vi "Dipper Fridge Resistance Measurement 1.1.vi"() -> ()   [LabVIEW 2011]
uses:
  <vilib>/express/express arith-compare/Formula/XNode/ExpressFormulaBlockNode.xnode
panel:
  out "Output Power":dbl[unit]
  out "Heater Power (%)":string
  in  "Save":bool
  out "var":i32
  in  "error in (no error) 2":errorcluster
  in  "Output Range":string(combo)
  in  "Heater Power (%)":dbl caption="y"
  out "Heater Type (in Ohm)":string
  out "Heater Current (in %)":string
  out "Heater":bool
  in  "Heater":bool
  out "Boolean":bool
  in  "Power":bool
  in  "Date format (0)":enum16{"short", "long", "abbreviated"}(ring)
  out "Lakeshore":cluster{dbl[], dbl[unit][]}(graph)
  out "Chanel A":cluster{dbl[], dbl[unit][]}(graph)
  out "size (in bytes)":i64
  out "Chanel B":cluster{dbl[], dbl[]}(graph)
  out "Warning":string="Can't be smaller than 1 s"
  in  "File Path":path
  out "current time":timestamp
  out "Number of Data points":i32
  in  "Time delay":u32
  in  "error in (no error)":errorcluster
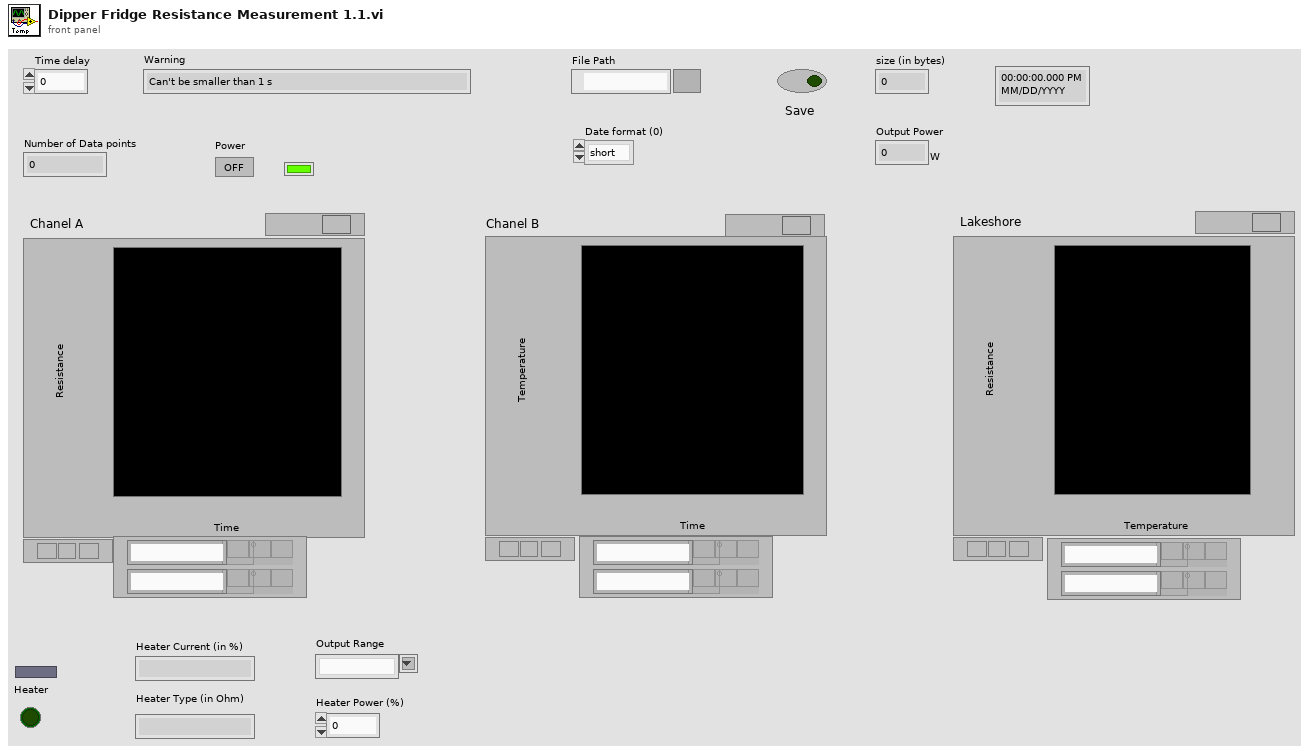
[diagram p1: front panel]
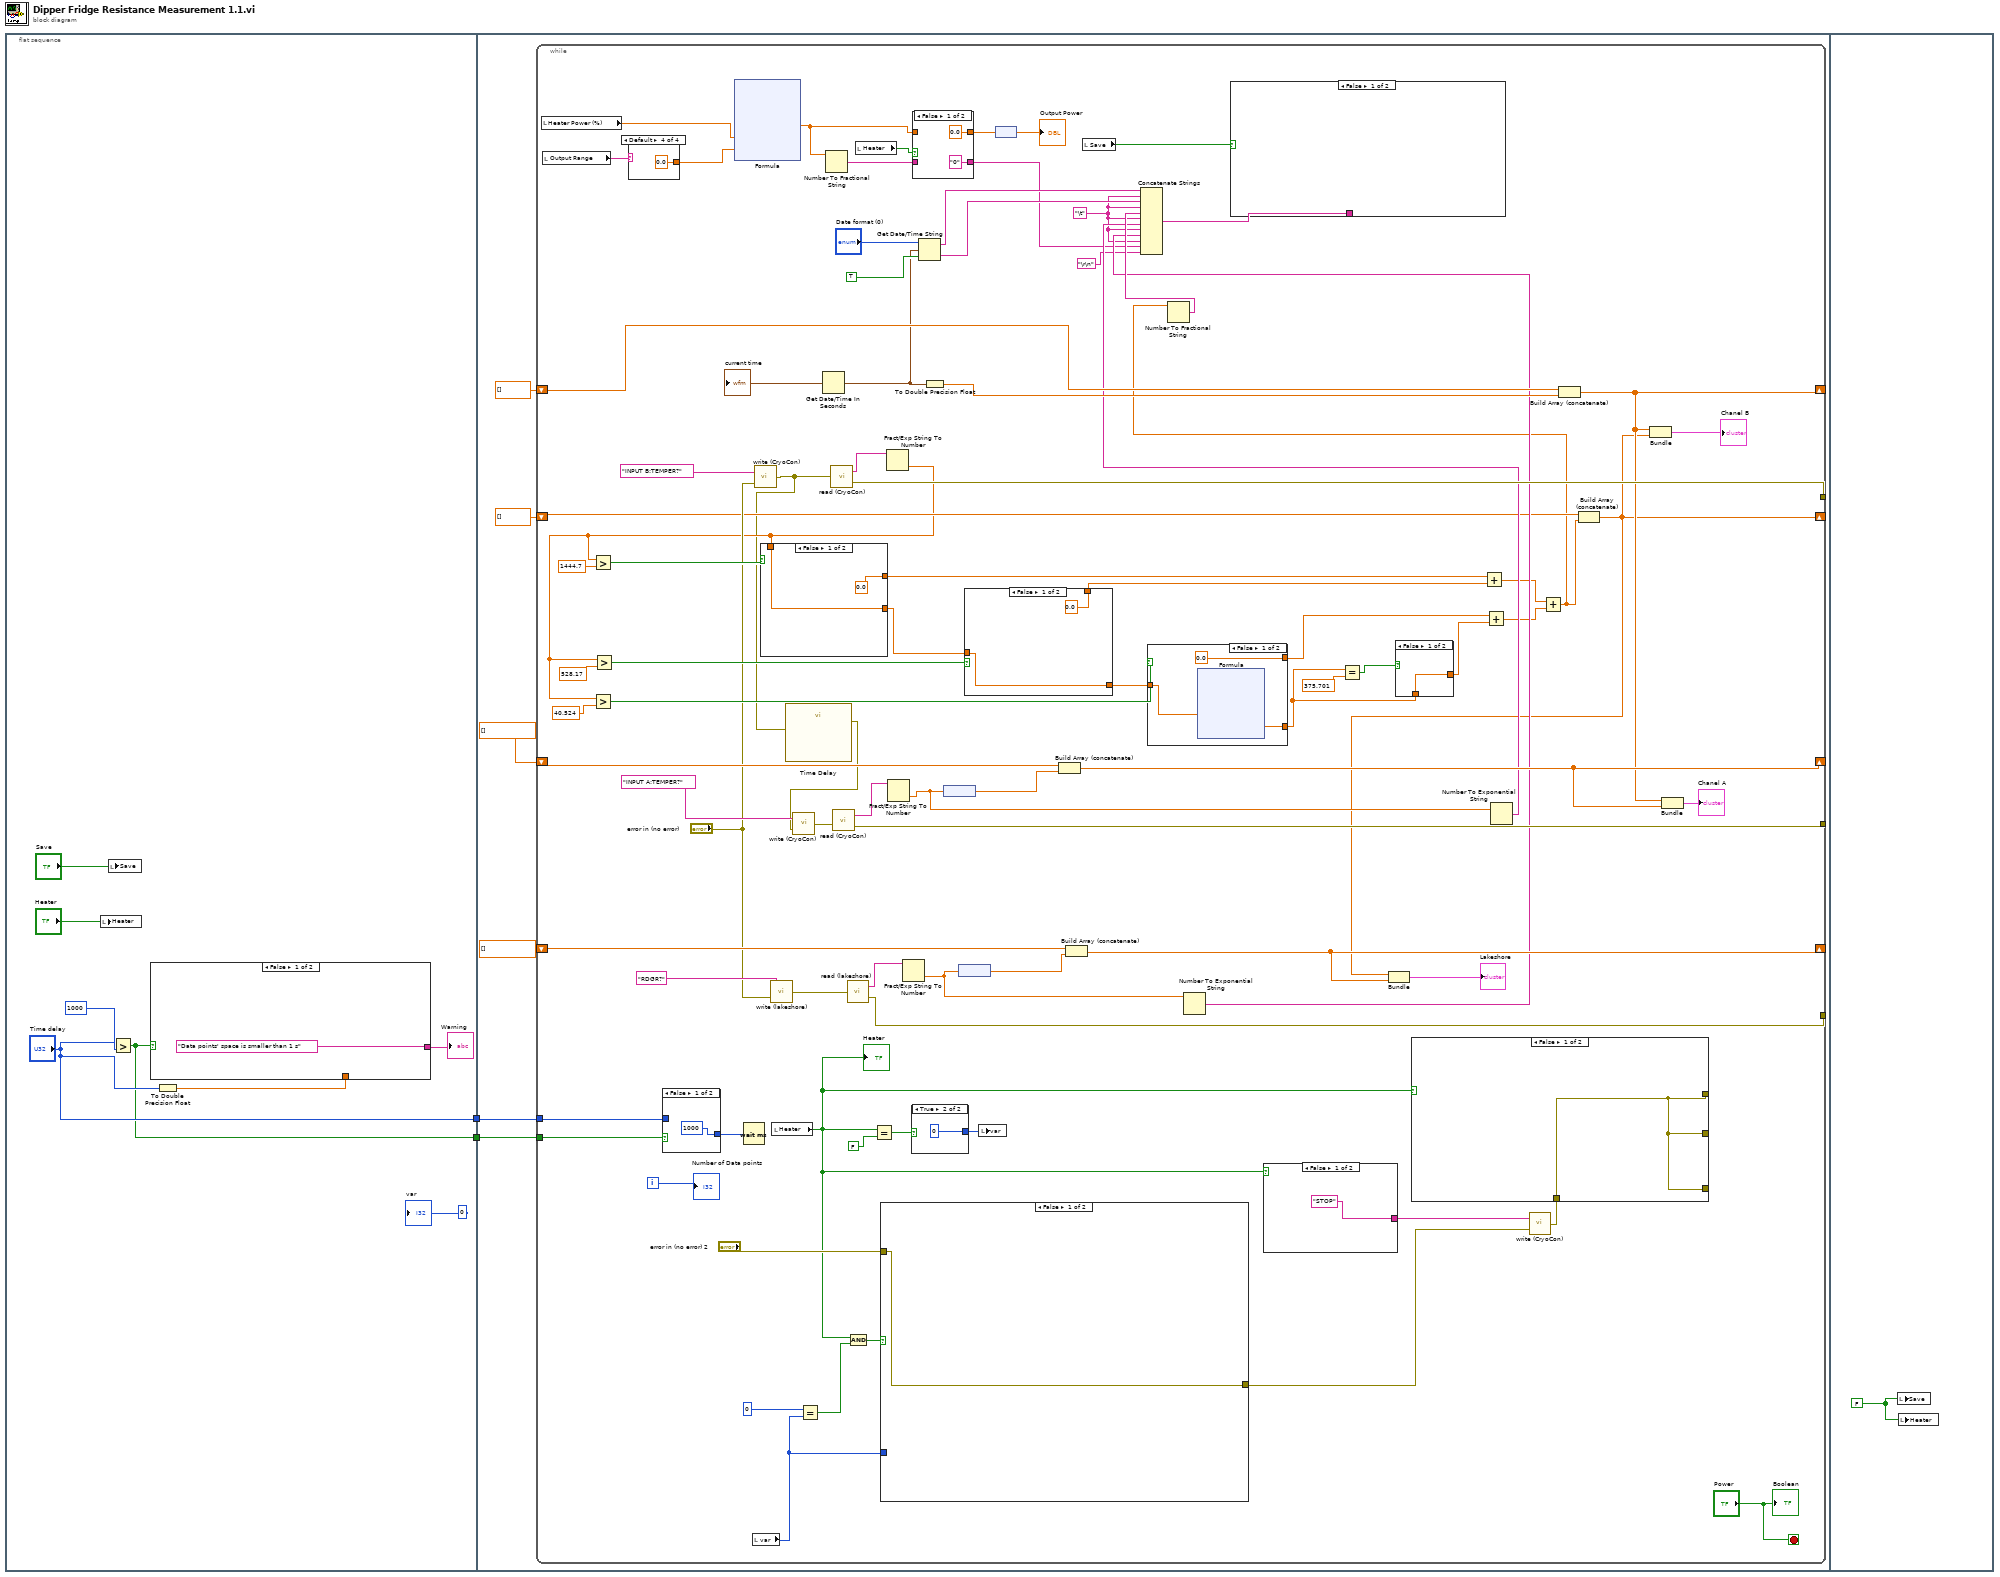
[diagram p0: block diagram]
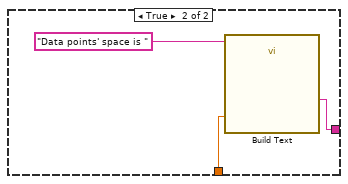
[diagram p2: hidden frame]
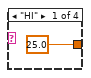
[diagram p4: hidden frame]
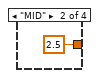
[diagram p5: hidden frame]
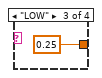
[diagram p6: hidden frame]
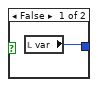
[diagram p7: hidden frame]
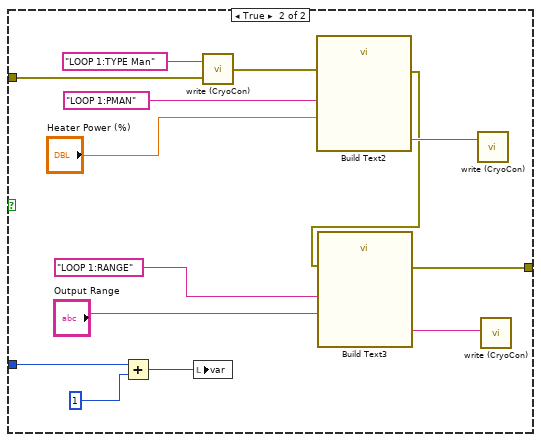
[diagram p8: hidden frame]
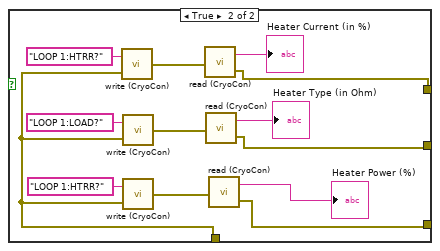
[diagram p9: hidden frame]
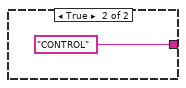
[diagram p10: hidden frame]
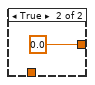
[diagram p11: hidden frame]
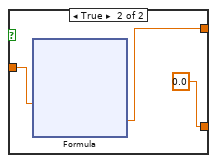
[diagram p12: hidden frame]
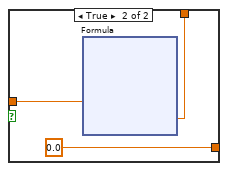
[diagram p13: hidden frame]
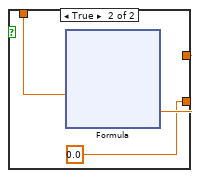
[diagram p14: hidden frame]
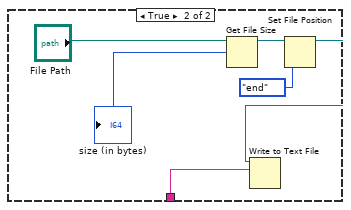
[diagram p16: hidden frame]
diagram:
  n1 = flat-sequence {
    tunnel: ["Time delay"] -> w2
    tunnel: [w5] -> w1
    tunnel: w2 -> [w20]
    tunnel: w1 -> [w19]
    frame #0 {
      n2 = local write "Heater"("Heater") -> ()
      n3 = local write "Save"("Save") -> ()
      n4 = Greater?(x="Time delay", y=u32 1000 ("x")) -> (0:w5:bool)
      n5 = To Double Precision Float(number="Time delay") -> (double precision float=w7:dbl)
      n6 = case shown="False" w5 {
        tunnel: w7 -> [_ w12]
        tunnel: ["Data points' space is smaller than 1 s" w14] -> w8
        frame False {
        }
        frame True {
          n7 = call "Build Text"("Beginning Text"="Data points' space is ", "Y"=w12) -> ("Result"=w14:string)  [unwired: 12 in, 1 out]
        }
      }
      "Warning" <- w8
      "var" <- 0 ("var")
    }
    frame #1 {
      n8 = while {
        tunnel: [w104] -> _
        tunnel: [w103] -> _
        tunnel: [w99] -> _
        shift-right: [w81] -> _
        shift-left: dbl[] [] -> [w94]
        tunnel: w20 -> [w93]
        tunnel: w19 -> [w92]
        shift-right: [w85] -> _
        shift-left: dbl[unit][] [] -> [w86]
        shift-right: [w82] -> _
        shift-left: dbl[unit][] [] -> [w83]
        shift-right: [w60] -> _
        shift-left: dbl[] [] -> [w63]
        i -> [w96]
        stop <- "Power" stop-if-true
        w38 = "\t"
        n9 = local read "Heater Power (%)"() -> (w33:dbl)
        n10 = local read "Output Range"() -> (w31:string)
        n11 = case shown="Default" w31 {
          tunnel: [25.0 ("X2") 2.5 ("X2") 0.25 ("X2") 0.0 ("X2")] -> w32
          frame "HI" {
          }
          frame "MID" {
          }
          frame "LOW" {
          }
          frame Default {
          }
        }
        n12 = case shown="False" w92 {
          tunnel: w93 -> [_ w210]
          tunnel: [1000 w210] -> w91
          frame False {
          }
          frame True {
          }
        }
        n13 = xnode "Formula"("X1"=w33, "X2"=w32) -> ("Result"=w25:dbl)  [unwired: 1 in, 1 out]
        n14 = Wait (ms)(milliseconds to wait=w91) -> ()  [unwired: 1 out]
        n15 = local read "var"() -> (w44:i32)
        n16 = call "write (CryoCon).vi"("error in (no error)"="error in (no error)", "write buffer"="INPUT B:TEMPER?") -> ("error out"=w22:errorcluster)
        n17 = call "write (lakeshore).vi"("error in (no error)"="error in (no error)", "write buffer"="RDGR?") -> ("error out"=w98:errorcluster)
        n18 = local read "Heater"() -> (w34:bool)
        "Heater" <- w34
        n19 = call "Time Delay"("error in (no error)"=w22) -> ("error out"=w21:errorcluster)  [unwired: 10 in]
        n20 = call "write (CryoCon).vi"("error in (no error)"=w21, "write buffer"="INPUT A:TEMPER?") -> ("error out"=w105:errorcluster)
        n21 = Equal?(x=0, y=w44) -> (x = y?=w42:bool)
        n22 = Get Date/Time In Seconds() -> (seconds since 1Jan1904=w90:timestamp)
        "current time" <- w90
        n23 = Number To Fractional String(number=w25) -> (F-format string=w29:string)  [unwired: 3 in]
        n24 = call "read (CryoCon).vi"("error in (no error)"=w22) -> ("read buffer"=w101:string, "error out"=w103:errorcluster)
        n25 = call "read (CryoCon).vi"("error in (no error)"=w105) -> ("read buffer"=w102:string, "error out"=w104:errorcluster)
        n26 = call "read (lakeshore).vi"("error in (no error)"=w98) -> ("read buffer"=w100:string, "error out"=w99:errorcluster)
        n27 = And(x=w34, y=w42) -> (x .and. y?=w41:bool)
        n28 = local read "Heater"() -> (w27:bool)
        n29 = Equal?(x=w34, y=FALSE ("Heater")) -> (x = y?=w36:bool)
        n30 = case shown="False" w41 {
          tunnel: [w128 w136] -> w40
          tunnel: "error in (no error) 2" -> [w128 w132]
          tunnel: w44 -> [_ w135]
          frame False {
          }
          frame True {
            n31 = Add(x=w135, y=1) -> (x+y=w133:i32)
            n32 = local write "var"(w133) -> ()
            n33 = call "write (CryoCon).vi"("error in (no error)"=w132, "write buffer"="LOOP 1:TYPE Man") -> ("error out"=w131:errorcluster)
            n34 = call "Build Text2"("x"="LOOP 1:PMAN" ("write buffer"), "y"="Heater Power (%)", "error in (no error)"=w131) -> ("Result"=w141:string, "error out"=w137:errorcluster)  [unwired: 11 in]
            n35 = call "Build Text3"("x"="LOOP 1:RANGE" ("write buffer"), "y"="Output Range", "error in (no error)"=w137) -> ("Result"=w138:string, "error out"=w136:errorcluster)  [unwired: 11 in]
            n36 = call "write (CryoCon).vi"("write buffer"=w141) -> ()  [unwired: 1 in, 1 out]
            n37 = call "write (CryoCon).vi"("write buffer"=w138) -> ()  [unwired: 1 in, 1 out]
          }
        }
        n38 = Fract/Exp String To Number(string=w101) -> (number=w23:dbl)  [unwired: 3 in, 1 out]
        n39 = Greater?(x=w23, y=1444.7) -> (0:w71:bool)
        n40 = Greater?(x=w23, y=40.524) -> (0:w68:bool)
        n41 = Greater?(x=w23, y=528.17) -> (0:w70:bool)
        n42 = case shown="False" w71 {
          tunnel: w23 -> [w196 w200]
          tunnel: [0.0 w199] -> w57
          tunnel: [w196 0.0] -> w54
          frame False {
          }
          frame True {
            n43 = xnode "Formula"("X1"=w200) -> ("Result"=w199:dbl)  [unwired: 1 in, 1 out]
          }
        }
        n44 = Fract/Exp String To Number(string=w102) -> (number=w79:dbl)  [unwired: 3 in, 1 out]
        n45 = Fract/Exp String To Number(string=w100) -> (number=w78:dbl)  [unwired: 3 in, 1 out]
        n46 = case shown="True" w36 {
          tunnel: [w116 0] -> w35
          frame False {
            n47 = local read "var"() -> (w116:i32)
          }
          frame True {
          }
        }
        n48 = case shown="False" w27 {
          tunnel: w29 -> [_ w111]
          tunnel: ["0" w111] -> w28
          tunnel: w25 -> [_ w110]
          tunnel: [0.0 ("Result") w110] -> w24
          frame False {
          }
          frame True {
          }
        }
        n49 = Get Date/Time String(date format (0)="Date format (0)", seconds (now)=w90, want seconds? (F)=TRUE) -> (date string=w77:string, time string=w76:string)
        n50 = To Double Precision Float(number=w90) -> (double precision float=w89:dbl)
        n51 = node(w79) -> (w87:dbl[unit])
        n52 = node(w78) -> (w62:dbl[unit])
        n53 = case shown="False" w70 {
          tunnel: [0.0 w187] -> w56
          tunnel: w54 -> [w183 w186]
          tunnel: [w183 0.0] -> w53
          frame False {
          }
          frame True {
            n54 = xnode "Formula"("X2"=w186) -> ("Result"=w187:dbl)  [unwired: 1 in, 1 out]
          }
        }
        n55 = local write "var"(w35) -> ()
        n56 = node(w24) -> (→"Output Power":dbl[unit])
        n57 = Build Array (concatenate)(w86, w87) -> (w85:dbl[unit][])
        n58 = Build Array (concatenate)(w83, w62) -> (w82:dbl[unit][])
        n59 = local read "Save"() -> (w39:bool)
        n60 = case shown="False" w68 {
          tunnel: [0.0 w174] -> w55
          tunnel: [w162 0.0] -> w49
          tunnel: w53 -> [w161 w172]
          frame False {
            n61 = xnode "Formula"("X4"=w161) -> ("Result"=w162:dbl)  [unwired: 1 in, 1 out]
          }
          frame True {
            n62 = xnode "Formula"("X3"=w172) -> ("Result"=w174:dbl)  [unwired: 1 in, 1 out]
          }
        }
        n63 = Number To Exponential String(number=w78) -> (E-format string=w73:string)  [unwired: 3 in]
        n64 = case shown="False" w34 {
          tunnel: ["STOP" ("write buffer") "CONTROL" ("write buffer")] -> w47
          frame False {
          }
          frame True {
          }
        }
        n65 = Equal?(x=w49, y=375.701) -> (x = y?=w52:bool)
        n66 = case shown="False" w52 {
          tunnel: [w159 0.0 ("y")] -> w50
          tunnel: w49 -> [w159 _]
          frame False {
          }
          frame True {
          }
        }
        n67 = Add(x=w57, y=w56) -> (x+y=w65:dbl)
        n68 = Add(x=w55, y=w50) -> (x+y=w64:dbl)
        n69 = Number To Exponential String(number=w79) -> (E-format string=w74:string)  [unwired: 3 in]
        n70 = call "write (CryoCon).vi"("error in (no error)"=w40, "write buffer"=w47) -> ("error out"=w46:errorcluster)
        n71 = case shown="False" w34 {
          tunnel: [w143 w150] -> _
          tunnel: [w143 w149] -> _
          tunnel: w46 -> [w143 w148]
          tunnel: [w143 w147] -> _
          frame False {
          }
          frame True {
            n72 = call "write (CryoCon).vi"("error in (no error)"=w148, "write buffer"="LOOP 1:HTRR?") -> ("error out"=w156:errorcluster)
            n73 = call "write (CryoCon).vi"("error in (no error)"=w148, "write buffer"="LOOP 1:LOAD?") -> ("error out"=w153:errorcluster)
            n74 = call "write (CryoCon).vi"("error in (no error)"=w148, "write buffer"="LOOP 1:HTRR?") -> ("error out"=w146:errorcluster)
            n75 = call "read (CryoCon).vi"("error in (no error)"=w156) -> ("read buffer"=→"Heater Current (in %)":string, "error out"=w150:errorcluster)
            n76 = call "read (CryoCon).vi"("error in (no error)"=w153) -> ("read buffer"=→"Heater Type (in Ohm)":string, "error out"=w149:errorcluster)
            n77 = call "read (CryoCon).vi"("error in (no error)"=w146) -> ("read buffer"=→"Heater Power (%)":string, "error out"=w147:errorcluster)
          }
        }
        n78 = Add(x=w65, y=w64) -> (x+y=w48:dbl)
        n79 = Number To Fractional String(number=w48) -> (F-format string=w75:string)  [unwired: 3 in]
        n80 = Concatenate Strings(w77, w38, w76, w38, w75, w38, w74, w38, w73, w38, w28, "\r\n") -> (w88:string)
        n81 = case shown="False" w39 {
          tunnel: w88 -> [_ w216]
          frame False {
          }
          frame True {
            n82 = Get File Size(file="File Path") -> (refnum out=w214:refnum<file>, size (in bytes)=→"size (in bytes)":i64)  [unwired: 1 in, 1 out]
            n83 = Set File Position(refnum=w214, from (0:start)=enum16{"start", "end", "current"}."end") -> (refnum out=w213:refnum<file>)  [unwired: 2 in, 1 out]
            n84 = Write to Text File(file (use dialog)=w213, text=w216) -> ()  [unwired: 2 in, 3 out]
          }
        }
        n85 = Build Array (concatenate)(w94, w89) -> (w81:dbl[])
        n86 = Build Array (concatenate)(w63, w48) -> (w60:dbl[])
        n87 = Bundle(w60, w82) -> (→"Lakeshore":cluster{dbl[], dbl[unit][]})  [unwired: 1 in]
        n88 = Bundle(w81, w60) -> (→"Chanel B":cluster{dbl[], dbl[]})  [unwired: 1 in]
        n89 = Bundle(w81, w85) -> (→"Chanel A":cluster{dbl[], dbl[unit][]})  [unwired: 1 in]
        "Number of Data points" <- w96
        "Boolean" <- "Power"
      }
    }
    frame #2 {
      w217 = FALSE ("Save")
      n90 = local write "Save"(w217) -> ()
      n91 = local write "Heater"(w217) -> ()
    }
  }
